vi "Get V and C.vi"(0 "configuration file path":path=path "C:/TDS/t230054-rf-mezz-fct-main/Configuration/InstrumentsConfig.ini", 1 "File Name":string="InstrumentsConfig.ini", 2 "Section":string="PS Power", 3 "error in (no error)":errorcluster) -> (7 "Voltage":dbl, 8 "Current":dbl, 10 "error out":errorcluster)   [LabVIEW 2023]
uses:
  <vilib>/Utility/config.llb/Read Key (Double).vi
  <vilib>/Utility/config.llb/NI_LVConfig.lvlib
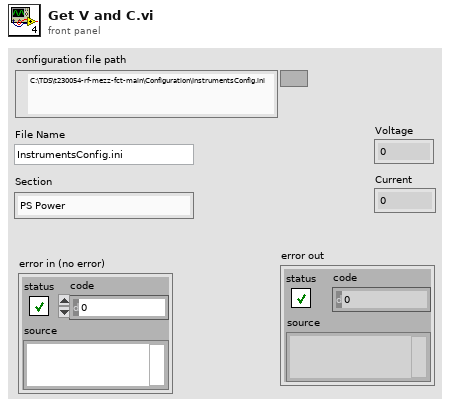
[diagram p1: front panel]
types:
  T1 = typedef "NI_LVConfig.lvlib/Config Data RefNum.ctl" = refnum<k1>
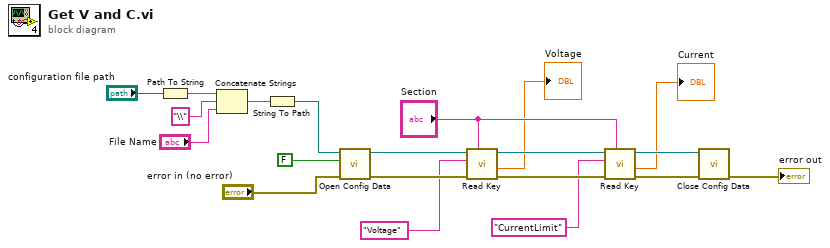
[diagram p0: block diagram]
diagram:
  n1 = Path To String(path="configuration file path") -> (string=w4:string)
  n2 = Concatenate Strings(w4, "\\" ("string"), "File Name") -> (w3:string)
  n3 = String To Path(string=w3) -> (path=w1:path)
  n4 = call <vilib>:"Open Config Data.vi"("error in (no error)"="error in (no error)", "create file if necessary (T)"=FALSE, "configuration file path"=w1) -> ("error out"=w14:errorcluster, "refnum"=w19:T1)  [unwired: 6 in, 1 out]
  n5 = call-poly <vilib>:"Read Key.vi"("section"="Section", "error in (no error)"=w14, "key"="Voltage", "refnum"=w19) -> ("error out"=w13:errorcluster, "value"=→"Voltage":dbl, "refnum out"=w18:T1)  [unwired: 4 in, 1 out]
  n6 = call-poly <vilib>:"Read Key.vi"("section"="Section", "error in (no error)"=w13, "key"="CurrentLimit", "refnum"=w18) -> ("error out"=w10:errorcluster, "value"=→"Current":dbl, "refnum out"=w17:T1)  [unwired: 4 in, 1 out]
  n7 = call <vilib>:"Close Config Data.vi"("error in (no error)"=w10, "refnum"=w17) -> ("error out"=→"error out":errorcluster)  [unwired: 8 in, 1 out]
